vi "Create CTR Encoder Channel.vi"(8 "error in (no error)":errorcluster, 9 "Physical channel":string, 10 "Name":string, 11 "Task in":refnum<k21>) -> (0 "error out":errorcluster, 2 "Encoder Channel Settings":string, 3 "Task out":refnum<k21>)   [LabVIEW 2021, in "Load Frame.lvlib"]
doc: "Create an Counter Input Encoder channel for 'Physical channel' with 'Name'."
uses:
  Load Frame.lvlib
  <vilib>/DAQmx/create/channels.llb/DAQmx Create Channel (CI-Position-Linear Encoder).vi
  <resource>/objmgr/daqmx.rc
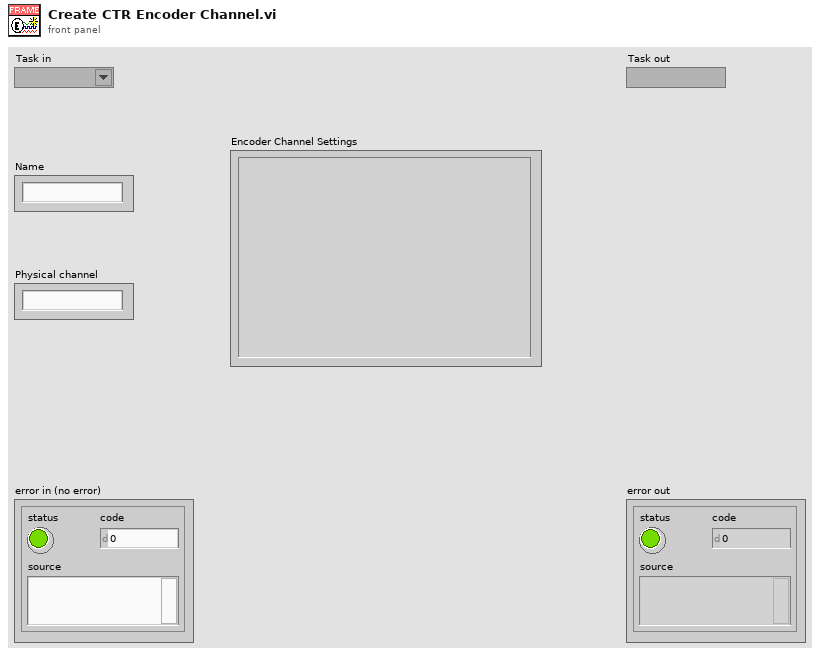
[diagram p1: front panel]
types:
  T1 = cluster{"Name":string, "Physical channel":string, "CI.Max":dbl, "CI.Min":dbl, "CI.MeasType":i32, "CI.Encoder.AInputTerm":string, "CI.Encoder.BInputTerm":string, "CI.Encoder.ZInputTerm":string, "CI.Encoder.ZIndexEnable":bool, "CI.Encoder.ZIndexVal":dbl, "CI.Encoder.ZIndexPhase":i32}
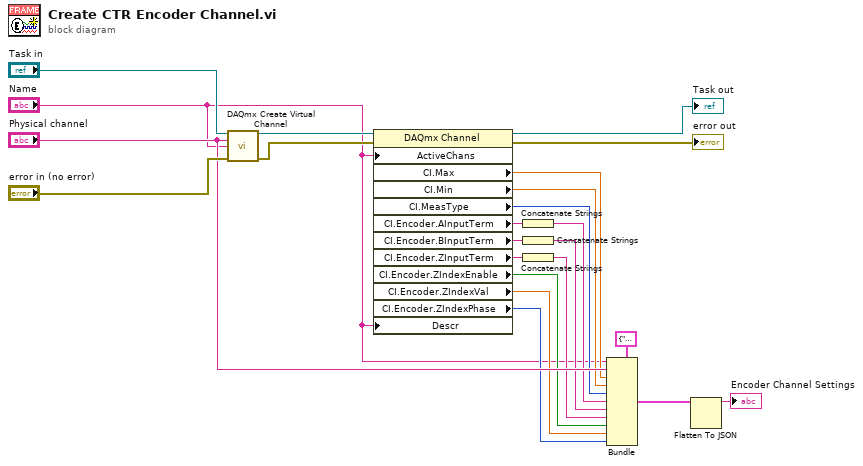
[diagram p0: block diagram]
diagram:
  n1 = call-poly <vilib>:"DAQmx Create Virtual Channel.vi"("task in"="Task in", "counter"="Physical channel", "name to assign"="Name", "error in"="error in (no error)") -> ("task out"=w22:refnum<k21>, "error out"=w19:errorcluster)  [unwired: 10 in]
  n2 = property class="DAQmx Channel"(reference=w22, error in=w19, "ActiveChans"="Name", "Descr"="Name") -> (reference out=→"Task out":refnum<k21>, error out=→"error out":errorcluster, "CI.Max"=w15:dbl, "CI.Min"=w14:dbl, "CI.MeasType"=w13:i32, "CI.Encoder.AInputTerm"=w12:tag, "CI.Encoder.BInputTerm"=w11:tag, "CI.Encoder.ZInputTerm"=w10:tag, "CI.Encoder.ZIndexEnable"=w9:bool, "CI.Encoder.ZIndexVal"=w8:dbl, "CI.Encoder.ZIndexPhase"=w7:i32)
  n3 = Concatenate Strings(w12) -> (w6:string)
  n4 = Concatenate Strings(w11) -> (w5:string)
  n5 = Concatenate Strings(w10) -> (w4:string)
  n6 = Bundle(cluster=T1 {"Name"="", "Physical channel"="", "CI.Max"=0.0, "CI.Min"=0.0, "CI.MeasType"=0, "CI.Encoder.AInputTerm"="", "CI.Encoder.BInputTerm"="", "CI.Encoder.ZInputTerm"="", "CI.Encoder.ZIndexEnable"=FALSE, "CI.Encoder.ZIndexVal"=0.0, "CI.Encoder.ZIndexPhase"=0} ("Encoder Channel Settings"), "Name"="Name", "Physical channel"="Physical channel", "CI.Max"=w15, "CI.Min"=w14, "CI.MeasType"=w13, "CI.Encoder.AInputTerm"=w6, "CI.Encoder.BInputTerm"=w5, "CI.Encoder.ZInputTerm"=w4, "CI.Encoder.ZIndexEnable"=w9, "CI.Encoder.ZIndexVal"=w8, "CI.Encoder.ZIndexPhase"=w7) -> (w3:T1)
  n7 = Flatten To JSON(anything=w3) -> (JSON string=→"Encoder Channel Settings":string)  [unwired: 2 in, 1 out]
